vi "signal generator.vi"() -> ()   [LabVIEW 2023]
uses:
  <vilib>/measure/NI_MABase.lvlib
panel:
  in  "amplitude 2":dbl=1.0 format="%0.2p"
  in  "frequency 2":dbl=10.0 format="%0.2p"
  in  "amplitude":dbl=1.0 format="%0.2p"
  in  "frequency":dbl=10.0 format="%0.2p"
  out "Waveform Chart":waveform(dbl)(graph)
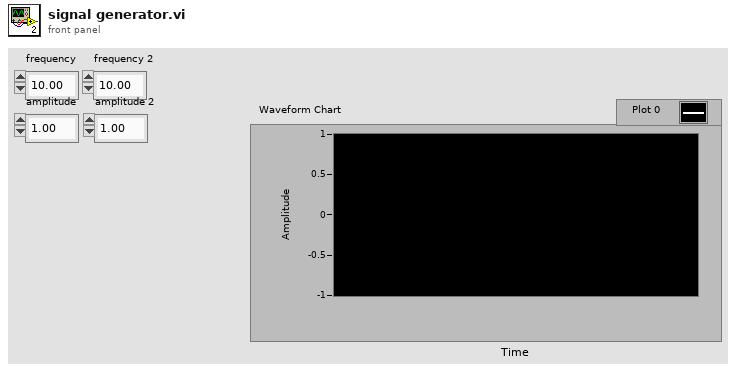
[diagram p1: front panel]
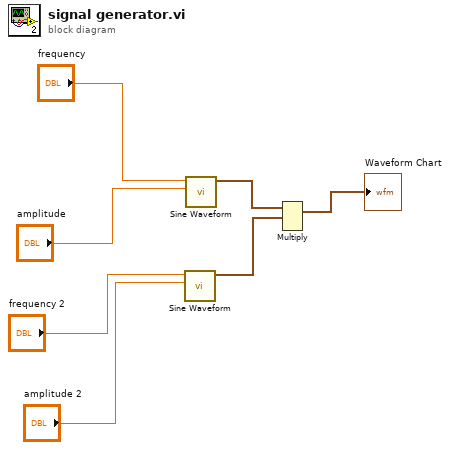
[diagram p0: block diagram]
diagram:
  n1 = call <vilib>:"Sine Waveform.vi"("amplitude"="amplitude 2", "frequency"="frequency 2") -> ("signal out"=w4:waveform(dbl))  [unwired: 8 in, 1 out]
  n2 = call <vilib>:"Sine Waveform.vi"("amplitude"="amplitude", "frequency"="frequency") -> ("signal out"=w5:waveform(dbl))  [unwired: 8 in, 1 out]
  n3 = Multiply(1:w4, 2:w5) -> (0:→"Waveform Chart":waveform(dbl))  [unwired: 1 in, 1 out]
